vi "Exit In Place Element Array.vi"(0 "Diagram in":refnum<vi>, 5 "Elements":refnum<vi>[](array[refnum]), 7 "Outputs":refnum<vi>[](array[refnum]), 11 "error in (no error)":errorcluster) -> (4 "Diagram out":refnum<vi>, 6 "Array":refnum<vi>, 8 "Indices":refnum<vi>[][](array[refnum]), 10 "Outputs":refnum<vi>[](array[refnum]), 15 "error out":errorcluster)   [LabVIEW 2015, in "Scripting.lvlib"]
doc: "Exits the In Place Element Structure that owns <B>Diagram in</B>, supplying the structure's owning diagram at <B>Diagram out</B>.\n\n<B>Elements</B> are the terminals to wire to the Replace Array Subset node's element terminals.\n\n<B>Array</B> is the array output terminal of the Replace Array Subset node.\n\n<B>Indices</B> are the index output terminals of the Replace Array Subset node."
uses:
  Scripting.lvlib
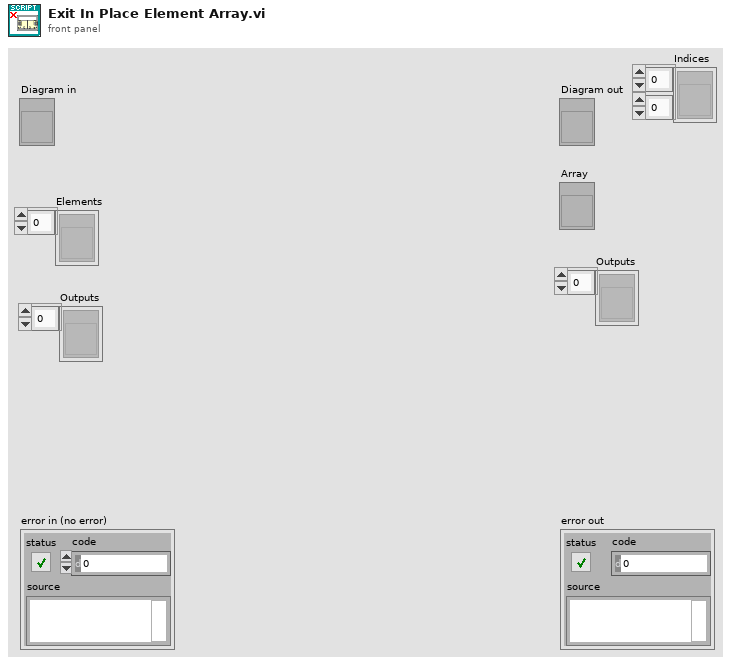
[diagram p1: front panel]
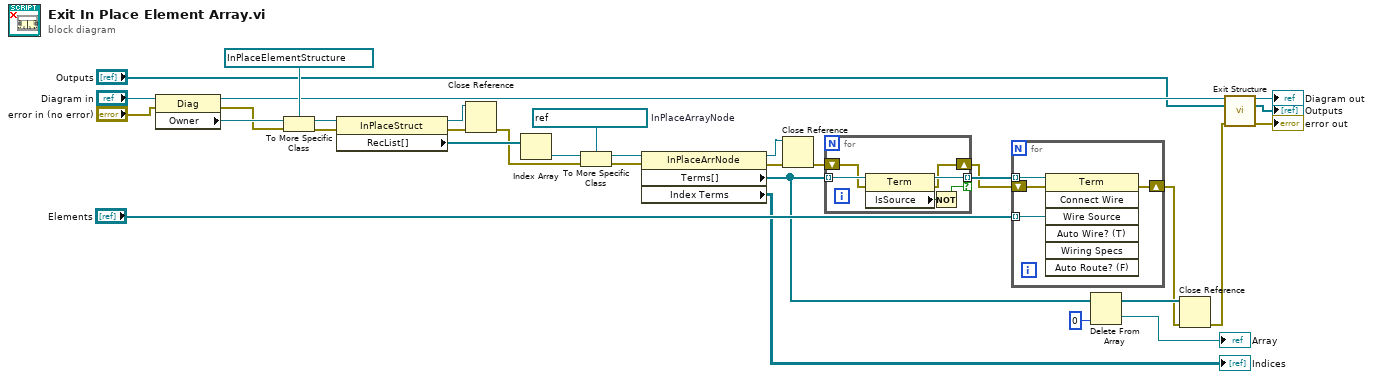
[diagram p0: block diagram]
diagram:
  w16 = refnum<vi> refnum  # InPlaceArrayNode
  n1 = property class="Diag"(reference="Diagram in", error in="error in (no error)") -> (reference out=w24:refnum<vi>, error out=w25:errorcluster, "Owner"=w33:refnum<vi>)
  n2 = To More Specific Class(target class=refnum<vi> refnum ("reference"), reference=w33, error in=w25) -> (specific class reference=w29:refnum<vi>, error out=w31:errorcluster)
  n3 = property class="InPlaceStruct"(reference=w29, error in=w31) -> (reference out=w7:refnum<vi>, error out=w32:errorcluster, "RecList[]"=w30:refnum<vi>[])
  n4 = Close Reference(reference=w7, error in (no error)=w32) -> (error out=w8:errorcluster)
  n5 = Index Array(array=w30) -> (element=w18:refnum<vi>)  [unwired: 1 in]
  n6 = To More Specific Class(target class=w16, reference=w18, error in=w8) -> (specific class reference=w17:refnum<vi>, error out=w19:errorcluster)
  n7 = property class="InPlaceArrNode"(reference=w17, error in=w19) -> (reference out=w5:refnum<vi>, error out=w11:errorcluster, "Terms[]"=w12:refnum<vi>[], "Index Terms"=→"Indices":refnum<vi>[][])
  n8 = Close Reference(reference=w5, error in (no error)=w11) -> (error out=w6:errorcluster)
  n9 = for {
    tunnel: w12 -> [w39] mode=indexing
    tunnel: [w38] -> w10 mode=indexing if=w36
    shift-right: [w34] -> w9
    shift-left: w6 -> [w35]
    n10 = property class="Term"(reference=w39, error in=w35) -> (reference out=w38:refnum<vi>, error out=w34:errorcluster, "IsSource"=w37:bool)
    n11 = Not(x=w37) -> (.not. x?=w36:bool)
  }
  n12 = for {
    tunnel: "Elements" -> [w42] mode=indexing
    shift-right: [w41] -> w2
    shift-left: w9 -> [w43]
    tunnel: w10 -> [w40] mode=indexing
    n13 = invoke class="Term" method="Connect Wire"(reference=w40, error in=w43, "Wire Source"=w42) -> (error out=w41:errorcluster)  [unwired: 4 in, 6 out]
  }
  n14 = Delete From Array(array=w12, index=0) -> (deleted portion=→"Array":refnum<vi>, array with subset deleted=w3:refnum<vi>[])  [unwired: 1 in]
  n15 = Close Reference(reference=w3, error in (no error)=w2) -> (error out=w1:errorcluster)
  n16 = call "Exit Structure.vi"("Diagram in"=w24, "Outputs"="Outputs", "error in (no error)"=w1) -> ("Diagram out"=→"Diagram out":refnum<vi>, "Outputs"=→"Outputs":refnum<vi>[], "error out"=→"error out":errorcluster)  [unwired: 10 in]
